vi "Debug Print.vi"(8 "error out":errorcluster, 9 "comment":string, 10 "Index":string, 11 "Module":string) -> ()   [LabVIEW 2020, in "Vires VTD Engine.lvlib"]
uses:
  Vires VTD Engine.lvlib
  <vilib>/NI VeriStand/Custom Device Tools/Custom Device Utility Library/Custom Device Utility Library.lvlib
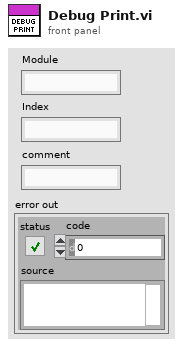
[diagram p1: front panel]
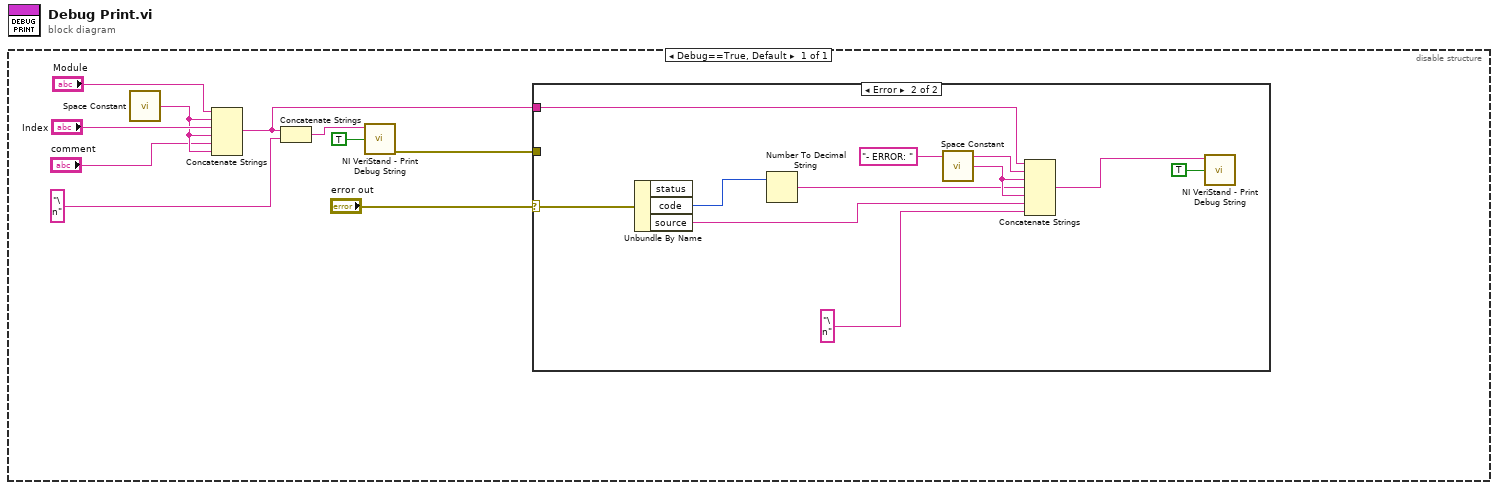
[diagram p0: block diagram]
diagram:
  n1 = disable-structure shown="Debug==True, Default" {
    frame condition #0 (active) {
      n2 = call <vilib>:"Space Constant.vi"() -> ("String"=w2:string)
      n3 = Concatenate Strings("Module", w2, "Index", w2, "comment", w2) -> (w3:string)
      n4 = Concatenate Strings(w3, "\n" ("Message")) -> (w4:string)
      n5 = call <vilib>:"NI VeriStand - Print Debug String.vi"("Add to log file? (F)"=TRUE ("Add to log file? (T)"), "Message"=w4) -> ("error out"=w8:errorcluster)  [unwired: 9 in]
      n6 = case shown="Error" "error out" {
        selector: "error out" -> [_ w18]
        tunnel: w8 -> [_ _]
        tunnel: w3 -> [_ w11]
        frame No Error {
        }
        frame Error {
          n7 = Unbundle By Name(w18) -> ("code"=w17:i32, "source"=w14:string)  [unwired: 1 out]
          n8 = Number To Decimal String(number=w17) -> (decimal integer string=w15:string)  [unwired: 1 in]
          n9 = call <vilib>:"Space Constant.vi"() -> ("String"=w19:string)
          n10 = Concatenate Strings(w11, "- ERROR: ", w19, w15, w19, w14, "\n" ("Message")) -> (w12:string)
          n11 = call <vilib>:"NI VeriStand - Print Debug String.vi"("Add to log file? (F)"=TRUE ("Add to log file? (T)"), "Message"=w12) -> ()  [unwired: 9 in, 1 out]
        }
      }
    }
  }
